vi "Create_New_Build.vi"(6 "buildSpecName":string, 7 "Programmatic? (false)":bool, 8 "error in (no error)":errorcluster, 9 "buildObject":T1, 10 "Destination Path":path, 11 "AB_WebService in":refnum<class "AB_WebService.lvclass">) -> (0 "error out":errorcluster, 3 "AB_WebService out":refnum<class "AB_WebService.lvclass">)   [LabVIEW 2020, in "AB_WebService.lvclass"]
uses:
  <vilib>/AppBuilder/AB_Classes/WebService/AB_WebService.lvclass
  e:/builds/penguin/labview/branches/2020/dev/dist/vi.lib/AppBuilder/AB_Classes/TargetFile/AB_Targetfile.lvclass
  e:/builds/penguin/labview/branches/2020/dev/dist/vi.lib/AppBuilder/AB_Classes/Build/AB_Build.lvclass
  <resource>/Framework/Providers/API/ItemRef.ctl
  <vilib>/AppBuilder/AB_LabelType.ctl
  <vilib>/AppBuilder/AB_Classes/WebService/AB_WebService.lvclass/AB_WebService.ctl
  <resource>/Framework/Providers/Common/provcom_StringGlobals.vi
  <vilib>/AppBuilder/AB_Classes/TargetFile/AB_Targetfile.lvclass
  <vilib>/AppBuilder/AB_Classes/Build/AB_Build.lvclass
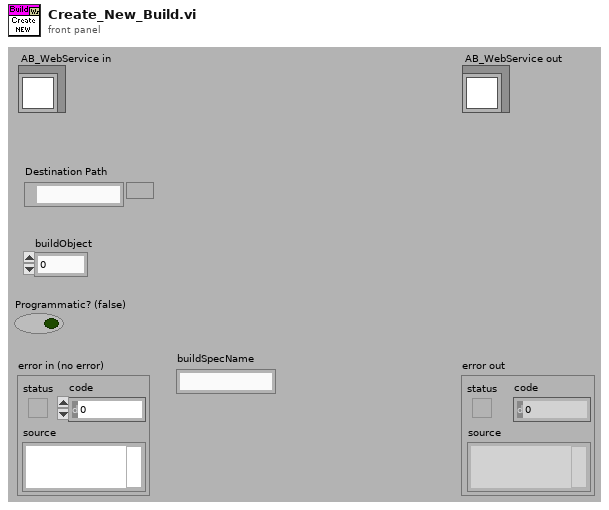
[diagram p1: front panel]
types:
  T1 = typedef "ItemRef.ctl" = u64
  T2 = typedef "AB_LabelType.ctl" = enum16{"buildSpec", "targetFilename"}
  T3 = typedef "AB_Targetfile.ctl" = cluster{"targetfileName":string, "targetfileGUID":string, "enableDebugging":bool, "versionInfo":cluster{"productName":string, "legalCopyright":string, "companyName":string, "internalName":string, "fileDescription":string}, "eng_consolidatedTypeInfo":string, "fastFileFormat":bool, "eng_LEIFBuildData":u32, "versionIndependent":bool}
  T4 = typedef "AB_Build.ctl" = cluster{"buildSpecName":string, "buildSpecDescription":string, "destinations":refnum<class "AB_Destination.lvclass">[], "exclusionOption":T5, "defaultLanguage":string, "supportedLanguages":string[], "excludedDirectories":path[], "buildContext":refnum<vi>, "buildObject":T1, "preview":bool, "programatic":bool, "progressBarEvents":T6, "userLog_Path":path, "preActionID":string, "preAction_Path":path, "postActionID":string, "postAction_Path":path, "eng_checkForBrokenVIs?":bool, "eng_verboseLinkerErrors?":bool, "localDest_Path":path, "targetDest_Path":path, "removeVIObject":u16, "cache":refnum<class "PreviewCache.lvclass">, "use cache":bool, "previewCache_ID":string, "buildCache_ID":string, "eng_TempLocalDest_Path":path, "eng_collectDependencies?":bool, "versionInfo":cluster{"buildVersion":cluster{"major":u16, "minor":u16, "patch":u16, "build":u16}, "autoIncrement":bool}, "eng_enableVIChecksums":bool}
  T5 = typedef "AB_Exclusion_Option.ctl" = cluster{"typedefs":bool, "polymorphicVIs":bool, "unusedLibraryItems":bool, "modifyLibraryFile":bool, "edit-timeDependencies":bool, "inlineVIs":bool, "dependent PPLs":bool, "dependent DLLs":bool}
  T6 = typedef "provcom_ProgressBar_Events.ctl" = cluster{"newJob":refnum<user-event>, "newItem":refnum<user-event>, "errorMsg":T7, "cancel":refnum<user-event>}
  T7 = typedef "mxLvBuildError.ctl" = refnum<user-event>
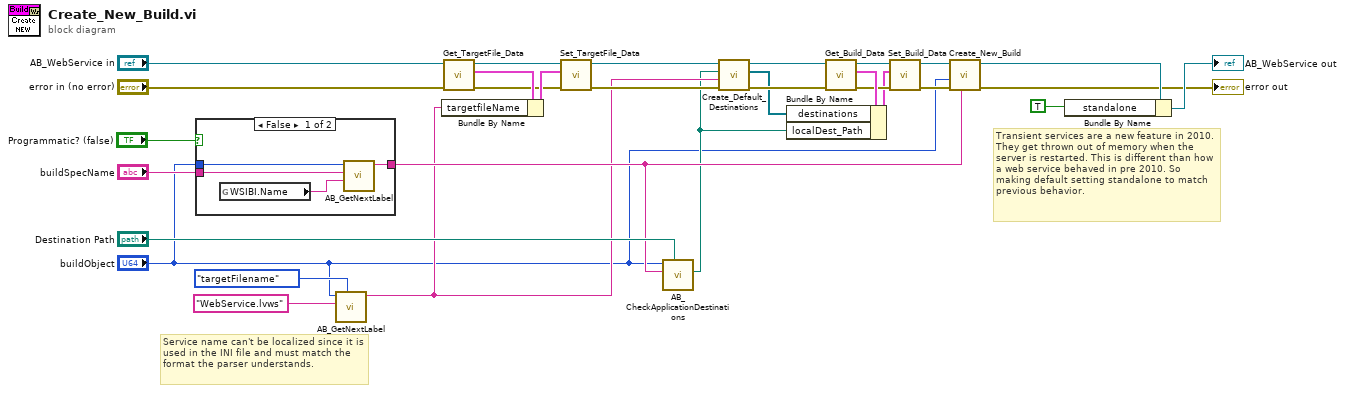
[diagram p0: block diagram]
diagram:
  # "Transient services are a new feature in 2010. They get thrown out of memory when the server is restarted. This is different than how a web service behaved in pre 2010. So making default setting standalone to match previous behavior."
  # "Service name can't be localized since it is used in the INI file and must match the format the parser understands."
  n1 = case shown="False" "Programmatic? (false)" {
    tunnel: "buildSpecName" -> [w32 w35]
    tunnel: [w34 w35] -> w22
    tunnel: "buildObject" -> [w31 _]
    frame False {
      n2 = global read "provcom_StringGlobals.vi" "WSIBI.Name"() -> (w33:string)
      n3 = call <vilib>:"AB_GetNextLabel.vi"("default name"=w33, "supplied name"=w32, "buildObject"=w31) -> ("New label"=w34:string)  [unwired: 2 in, 6 out]
    }
    frame True {
    }
  }
  n4 = call <vilib>:"AB_GetNextLabel.vi"("label type (buildSpec)"=AB_LabelType."targetFilename", "supplied name"="WebService.lvws" ("Default name"), "buildObject"="buildObject") -> ("New label"=w8:string)  [unwired: 2 in, 6 out]
  n5 = call <vilib>:"Get_TargetFile_Data.vi"("error in (no error)"="error in (no error)", "AB_Targetfile in"="AB_WebService in") -> ("error out"=w14:errorcluster, "data"=w16:T3, "AB_Targetfile out"=w9:refnum<class "AB_WebService.lvclass">)  [unwired: 7 in]
  n6 = Bundle By Name(cluster=w16, "targetfileName"=w8) -> (w15:T3)
  n7 = call <vilib>:"Set_TargetFile_Data.vi"("error in (no error)"=w14, "data"=w15, "AB_Targetfile in"=w9) -> ("error out"=w10:errorcluster, "AB_Targetfile out"=w11:refnum<class "AB_WebService.lvclass">)  [unwired: 7 in]
  n8 = call <vilib>:"AB_CheckApplicationDestinations.vi"("Destination Path"="Destination Path", "buildSpecName"=w22, "buildObject"="buildObject") -> ("Checked base path"=w7:path)  [unwired: 2 in, 6 out]
  n9 = call-dynamic "Create_Default_Destinations.vi"("error in (no error)"=w10, "Destination Name"=w8, "Destination Path"=w7, "AB_WebService in"=w11) -> ("error out"=w18:errorcluster, "default dests"=w17:refnum<class "AB_Destination.lvclass">[], "AB_WebService out"=w19:refnum<class "AB_WebService.lvclass">)  [unwired: 5 out]
  n10 = call <vilib>:"Get_Build_Data.vi"("error in (no error)"=w18, "Class in"=w19) -> ("error out"=w27:errorcluster, "data"=w29:T4, "Class out"=w28:refnum<class "AB_WebService.lvclass">)  [unwired: 7 out]
  n11 = Bundle By Name(cluster=w29, "destinations"=w17, "localDest_Path"=w7) -> (w26:T4)
  n12 = call <vilib>:"Set_Build_Data.vi"("error in (no error)"=w27, "data"=w26, "Class in"=w28) -> ("error out"=w23:errorcluster, "Class out"=w24:refnum<class "AB_WebService.lvclass">)  [unwired: 7 out]
  n13 = call-parent "Create_New_Build.vi"("buildSpecName"=w22, "error in (no error)"=w23, "buildObject"="buildObject", "AB_Targetfile in"=w24) -> ("error out"=→"error out":errorcluster, "AB_Targetfile out"=w2:refnum<class "AB_WebService.lvclass">)  [unwired: 2 in, 4 out]
  n14 = Bundle By Name(cluster=w2, "standalone"=TRUE ("data.standalone")) -> (→"AB_WebService out":refnum<class "AB_WebService.lvclass">)
